vi "AFE_SGL_src.vi"(4 "ManualControl":T2, 5 "Range":T5={"PLL_PIRad_high"=inf, "PLL_PiRad_low"=inf, "IQcmd_high"=inf, "IQcmd_low"=inf, "IDcmd_high"=inf, "IDcmd_low"=inf, "VDcmd_high"=inf, "VDcmd_low"=inf, "VQmcd_high"=inf, "VQcmd_low"=inf}, 6 "Parameters":T8, 7 "Gains":T6, 9 "Signals":T1, 10 "Setpoints":T7, 11 "Inputs":T9) -> (0 "Actions":T4, 3 "Outputs":T3)   [LabVIEW 2017]
uses:
  AFE/Inputs.ctl
  AFE/Parameters.ctl
  AFE/Setpoint.ctl
  AFE/Gains.ctl
  AFE/Range.ctl
  AFE/Actions.ctl
  AFE/Outputs.ctl
  AFE/ManualControl.ctl
  AFE/Signals.ctl
  AFE/CascadeControlSetpt.ctl
  AFE/CascadeControlProcVar.ctl
  <vilib>/rvi/Analysis/control/PID/Typedef/niFpgaPID_PIGains.ctl
  AFE/CascadeControlGains.ctl
  <vilib>/rvi/Analysis/control/PID/Typedef/niFpgaPID_OutputRange.ctl
  AFE/CascadeControlRange.ctl
  <vilib>/NI/PowerElectronicsControl/Transforms/_IPBuilder/AlphaBetaAndDQ_variants/ABCtoDQ_noSine_3PhasePowerInvariant_src.vi
  <vilib>/NI/PowerElectronicsControl/Transforms/_IPBuilder/AlphaBetaAndDQ_variants/DQtoABC_noSine_PowerInvariant_src.vi
  AFE/ActiveFrontEnd.lvlib
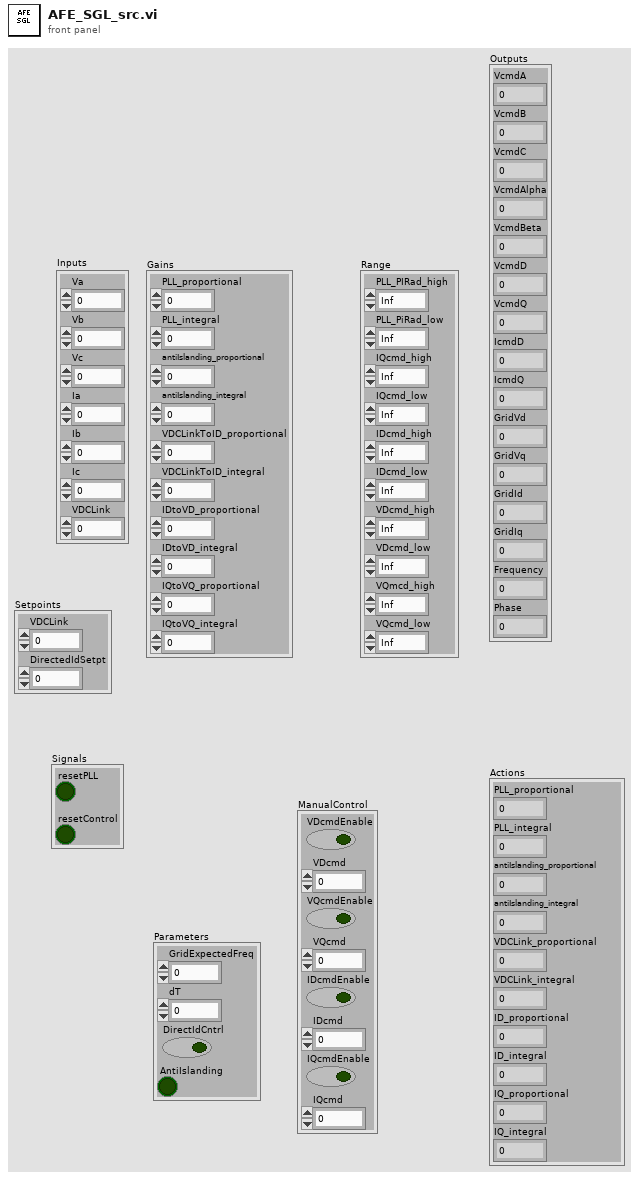
[diagram p1: front panel]
types:
  T1 = typedef "ActiveFrontEnd.lvlib/Signals.ctl" = cluster{"resetPLL":bool, "resetControl":bool}
  T2 = typedef "ActiveFrontEnd.lvlib/ManualControl.ctl" = cluster{"VDcmdEnable":bool, "VDcmd":sgl, "VQcmdEnable":bool, "VQcmd":sgl, "IDcmdEnable":bool, "IDcmd":sgl, "IQcmdEnable":bool, "IQcmd":sgl}
  T3 = typedef "ActiveFrontEnd.lvlib/Outputs.ctl" = cluster{"VcmdA":sgl, "VcmdB":sgl, "VcmdC":sgl, "VcmdAlpha":sgl, "VcmdBeta":sgl, "VcmdD":sgl, "VcmdQ":sgl, "IcmdD":sgl, "IcmdQ":sgl, "GridVd":sgl, "GridVq":sgl, "GridId":sgl, "GridIq":sgl, "Frequency":sgl, "Phase":sgl}
  T4 = typedef "ActiveFrontEnd.lvlib/Actions.ctl" = cluster{"PLL_proportional":sgl, "PLL_integral":sgl, "antiIslanding_proportional":sgl, "antiIslanding_integral":sgl, "VDCLink_proportional":sgl, "VDCLink_integral":sgl, "ID_proportional":sgl, "ID_integral":sgl, "IQ_proportional":sgl, "IQ_integral":sgl}
  T5 = typedef "ActiveFrontEnd.lvlib/Range.ctl" = cluster{"PLL_PIRad_high":sgl, "PLL_PiRad_low":sgl, "IQcmd_high":sgl, "IQcmd_low":sgl, "IDcmd_high":sgl, "IDcmd_low":sgl, "VDcmd_high":sgl, "VDcmd_low":sgl, "VQmcd_high":sgl, "VQcmd_low":sgl}
  T6 = typedef "ActiveFrontEnd.lvlib/Gains.ctl" = cluster{"PLL_proportional":sgl, "PLL_integral":sgl, "antiIslanding_proportional":sgl, "antiIslanding_integral":sgl, "VDCLinkToID_proportional":sgl, "VDCLinkToID_integral":sgl, "IDtoVD_proportional":sgl, "IDtoVD_integral":sgl, "IQtoVQ_proportional":sgl, "IQtoVQ_integral":sgl}
  T7 = typedef "ActiveFrontEnd.lvlib/Setpoint.ctl" = cluster{"VDCLink":sgl, "DirectedIdSetpt":sgl}
  T8 = typedef "ActiveFrontEnd.lvlib/Parameters.ctl" = cluster{"GridExpectedFreq":sgl, "dT":sgl, "DirectIdCntrl":bool, "AntiIslanding":bool}
  T9 = typedef "ActiveFrontEnd.lvlib/Inputs.ctl" = cluster{"Va":sgl, "Vb":sgl, "Vc":sgl, "Ia":sgl, "Ib":sgl, "Ic":sgl, "VDCLink":sgl}
  T10 = typedef "CascadeControlRange.ctl" = cluster{"antiIslanding_high":sgl, "antiIslanding_low":sgl, "VDCLink_high":sgl, "VDCLink_low":sgl, "ID_high":sgl, "ID_low":sgl, "IQ_high":sgl, "IQ_low":sgl}
  T11 = typedef "niFpgaPID_OutputRange.ctl" = cluster{"output high (Inf)":sgl, "output low (-Inf)":sgl}
  T12 = typedef "CascadeControlGains.ctl" = cluster{"antiIslanding_proportional":sgl, "antiIslanding_integral":sgl, "VDCLink_proportional":sgl, "VDCLink_integral":sgl, "ID_proportional":sgl, "ID_integral":sgl, "IQ_proportional":sgl, "IQ_integral":sgl}
  T13 = typedef "niFpgaPID_PIGains.ctl" = cluster{"proportional gain":sgl, "integral gain":sgl}
  T14 = typedef "CascadeControlProcVar.ctl" = cluster{"GridFrequency":sgl, "VDCLink":sgl, "GridId":sgl, "GridIq":sgl}
  T15 = typedef "CascadeControlSetpt.ctl" = cluster{"GridExpectedFreq":sgl, "VDCLink":sgl, "DirectedIdSetpt":sgl}
  T16 = typedef "ThreePhasePLLState.ctl" = cluster{"Phase":sgl}
  T17 = typedef "niFpgaPID_PIActions.ctl" = cluster{"proportional action":sgl, "integral action":sgl}
  T18 = typedef "CascadeControlAction.ctl" = cluster{"antiIslanding_proportional":sgl, "antiIslanding_integral":sgl, "VDCLink_proportional":sgl, "VDCLink_integral":sgl, "ID_proportional":sgl, "ID_integral":sgl, "IQ_proportional":sgl, "IQ_integral":sgl}
  T19 = typedef "ActiveFrontEnd.lvlib/DQ.ctl" = cluster{"D":sgl, "Q":sgl}
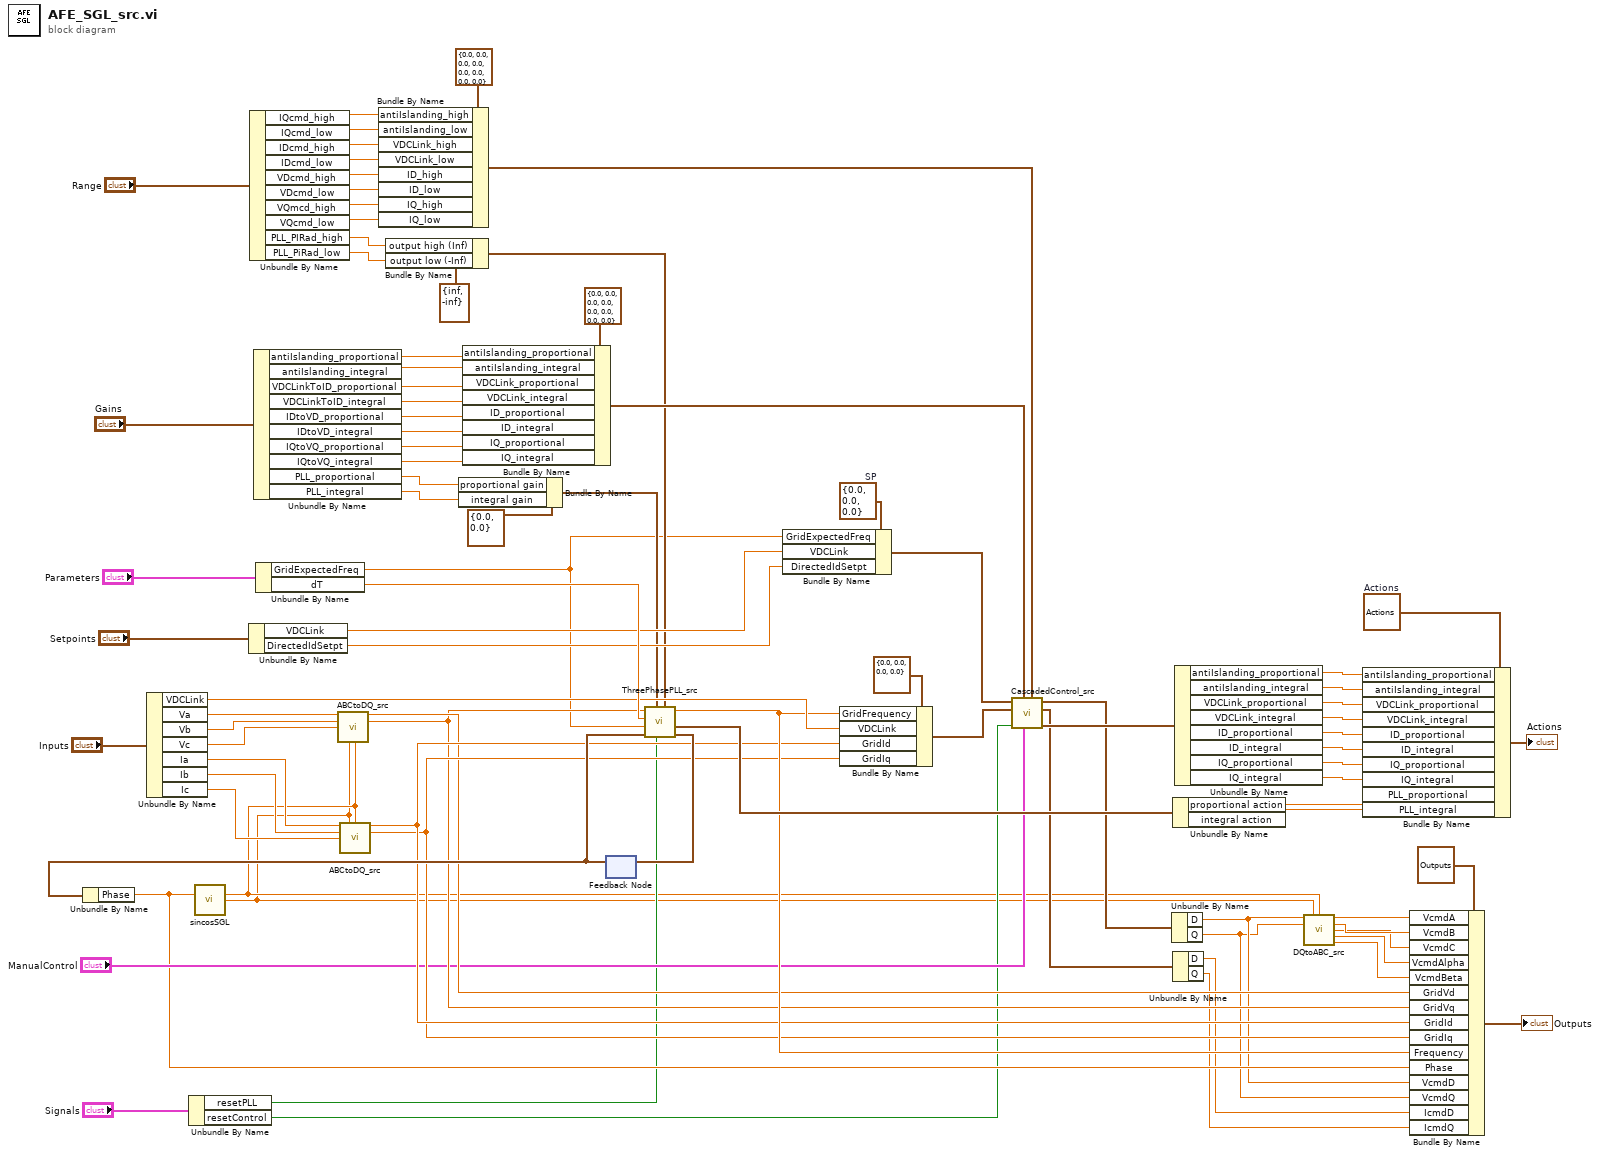
[diagram p0: block diagram]
diagram:
  w44 = T4 {"PLL_proportional"=0.0, "PLL_integral"=0.0, "antiIslanding_proportional"=0.0, "antiIslanding_integral"=0.0, "VDCLink_proportional"=0.0, "VDCLink_integral"=0.0, "ID_proportional"=0.0, "ID_integral"=0.0, "IQ_proportional"=0.0, "IQ_integral"=0.0}  # Actions
  w84 = T15 {"GridExpectedFreq"=0.0, "VDCLink"=0.0, "DirectedIdSetpt"=0.0}  # SP
  n1 = Unbundle By Name("Inputs") -> ("VDCLink"=w79:sgl, "Va"=w17:sgl, "Vb"=w16:sgl, "Vc"=w5:sgl, "Ia"=w89:sgl, "Ib"=w88:sgl, "Ic"=w6:sgl)
  n2 = Unbundle By Name("Signals") -> ("resetPLL"=w14:bool, "resetControl"=w13:bool)
  n3 = Unbundle By Name("Setpoints") -> ("VDCLink"=w77:sgl, "DirectedIdSetpt"=w76:sgl)
  n4 = Unbundle By Name("Range") -> ("IQcmd_high"=w54:sgl, "IQcmd_low"=w53:sgl, "IDcmd_high"=w52:sgl, "IDcmd_low"=w51:sgl, "VDcmd_high"=w50:sgl, "VDcmd_low"=w49:sgl, "VQmcd_high"=w48:sgl, "VQcmd_low"=w47:sgl, "PLL_PIRad_high"=w56:sgl, "PLL_PiRad_low"=w57:sgl)
  n5 = Unbundle By Name("Gains") -> ("antiIslanding_proportional"=w68:sgl, "antiIslanding_integral"=w67:sgl, "VDCLinkToID_proportional"=w66:sgl, "VDCLinkToID_integral"=w65:sgl, "IDtoVD_proportional"=w64:sgl, "IDtoVD_integral"=w63:sgl, "IQtoVQ_proportional"=w62:sgl, "IQtoVQ_integral"=w61:sgl, "PLL_proportional"=w71:sgl, "PLL_integral"=w70:sgl)
  n6 = Unbundle By Name("Parameters") -> ("GridExpectedFreq"=w19:sgl, "dT"=w81:sgl)
  n7 = Bundle By Name(cluster=T10 {"antiIslanding_high"=0.0, "antiIslanding_low"=0.0, "VDCLink_high"=0.0, "VDCLink_low"=0.0, "ID_high"=0.0, "ID_low"=0.0, "IQ_high"=0.0, "IQ_low"=0.0} ("Range"), "antiIslanding_high"=w54, "antiIslanding_low"=w53, "VDCLink_high"=w52, "VDCLink_low"=w51, "ID_high"=w50, "ID_low"=w49, "IQ_high"=w48, "IQ_low"=w47) -> (w46:T10)
  n8 = Bundle By Name(cluster=T11 {"output high (Inf)"=inf, "output low (-Inf)"=-inf} ("PLLrange"), "output high (Inf)"=w56, "output low (-Inf)"=w57) -> (w45:T11)
  n9 = Bundle By Name(cluster=T13 {"proportional gain"=0.0, "integral gain"=0.0} ("PLLgains"), "proportional gain"=w71, "integral gain"=w70) -> (w73:T13)
  n10 = Bundle By Name(cluster=T12 {"antiIslanding_proportional"=0.0, "antiIslanding_integral"=0.0, "VDCLink_proportional"=0.0, "VDCLink_integral"=0.0, "ID_proportional"=0.0, "ID_integral"=0.0, "IQ_proportional"=0.0, "IQ_integral"=0.0} ("Gains"), "antiIslanding_proportional"=w68, "antiIslanding_integral"=w67, "VDCLink_proportional"=w66, "VDCLink_integral"=w65, "ID_proportional"=w64, "ID_integral"=w63, "IQ_proportional"=w62, "IQ_integral"=w61) -> (w60:T12)
  n11 = feedback #1() -> (w85:T16)  [unwired: 1 in]
  n12 = Unbundle By Name(w85) -> ("Phase"=w18:sgl)
  n13 = call <vilib>:"sincosSGL.vi"("x"=w18) -> ("sinx"=w4:sgl, "cosx"=w3:sgl)  [unwired: 13 in]
  n14 = call-poly <vilib>:"ABCtoDQ_src.vi"("A"=w17, "cosx"=w3, "sinx"=w4, "B"=w16, "C"=w5) -> ("direct"=w22:sgl, "quadrature"=w21:sgl)  [unwired: 7 in, 2 out]
  n15 = call-poly <vilib>:"ABCtoDQ_src.vi"("A"=w89, "cosx"=w3, "sinx"=w4, "B"=w88, "C"=w6) -> ("direct"=w24:sgl, "quadrature"=w23:sgl)  [unwired: 7 in, 2 out]
  n16 = call "ThreePhasePLL_src.vi"("PLLrange"=w45, "reset"=w14, "PLLgains"=w73, "StateIn"=w85, "GridExpectedFreq"=w19, "dT"=w81, "Vq"=w21) -> ("StateOut"=w86:T16, "PLLactions"=w34:T17, "gridFrequency"=w25:sgl)  [unwired: 2 in]
  n17 = feedback-in #1(w86) -> ()
  n18 = Bundle By Name(cluster=w84, "GridExpectedFreq"=w19, "VDCLink"=w77, "DirectedIdSetpt"=w76) -> (w83:T15)
  n19 = Bundle By Name(cluster=T14 {"GridFrequency"=0.0, "VDCLink"=0.0, "GridId"=0.0, "GridIq"=0.0} ("PV"), "GridFrequency"=w25, "VDCLink"=w79, "GridId"=w24, "GridIq"=w23) -> (w75:T14)
  n20 = call "CascadedControl_src.vi"("Range"=w46, "ManualControl"="ManualControl", "Gains"=w60, "reset"=w13, "PV"=w75, "SP"=w83) -> ("Actions"=w43:T18, "Icmd"=w11:T19, "Vcmd"=w12:T19)  [unwired: 3 in]
  n21 = Unbundle By Name(w12) -> ("D"=w10:sgl, "Q"=w9:sgl)
  n22 = Unbundle By Name(w34) -> ("proportional action"=w33:sgl, "integral action"=w32:sgl)
  n23 = Unbundle By Name(w11) -> ("D"=w8:sgl, "Q"=w7:sgl)
  n24 = Unbundle By Name(w43) -> ("antiIslanding_proportional"=w42:sgl, "antiIslanding_integral"=w41:sgl, "VDCLink_proportional"=w40:sgl, "VDCLink_integral"=w39:sgl, "ID_proportional"=w38:sgl, "ID_integral"=w37:sgl, "IQ_proportional"=w36:sgl, "IQ_integral"=w35:sgl)
  n25 = call-poly <vilib>:"DQtoABC_src.vi"("direct"=w10, "cosx"=w3, "sinx"=w4, "quadrature"=w9) -> ("A"=w29:sgl, "B"=w28:sgl, "C"=w2:sgl, "alpha"=w1:sgl, "beta"=w27:sgl)  [unwired: 7 in]
  n26 = Bundle By Name(cluster=w44, "antiIslanding_proportional"=w42, "antiIslanding_integral"=w41, "VDCLink_proportional"=w40, "VDCLink_integral"=w39, "ID_proportional"=w38, "ID_integral"=w37, "IQ_proportional"=w36, "IQ_integral"=w35, "PLL_proportional"=w33, "PLL_integral"=w32) -> (→"Actions":T4)
  n27 = Bundle By Name(cluster=T3 {"VcmdA"=0.0, "VcmdB"=0.0, "VcmdC"=0.0, "VcmdAlpha"=0.0, "VcmdBeta"=0.0, "VcmdD"=0.0, "VcmdQ"=0.0, "IcmdD"=0.0, "IcmdQ"=0.0, "GridVd"=0.0, "GridVq"=0.0, "GridId"=0.0, "GridIq"=0.0, "Frequency"=0.0, "Phase"=0.0} ("Outpus"), "VcmdA"=w29, "VcmdB"=w28, "VcmdC"=w2, "VcmdAlpha"=w1, "VcmdBeta"=w27, "GridVd"=w22, "GridVq"=w21, "GridId"=w24, "GridIq"=w23, "Frequency"=w25, "Phase"=w18, "VcmdD"=w10, "VcmdQ"=w9, "IcmdD"=w8, "IcmdQ"=w7) -> (→"Outputs":T3)
